vi "EXCEL 画曲线.vi"(8 "错误输入（无错误）":errorcluster, 11 "路径":path) -> (0 "error IO":errorcluster, 1 "打开时间":u32, 2 "XY图":cluster{"X":dbl, "Y":dbl}[](graph), 3 "XY图 2":cluster{"X":dbl, "Y":dbl}[](array[cluster]))   [LabVIEW 2018]
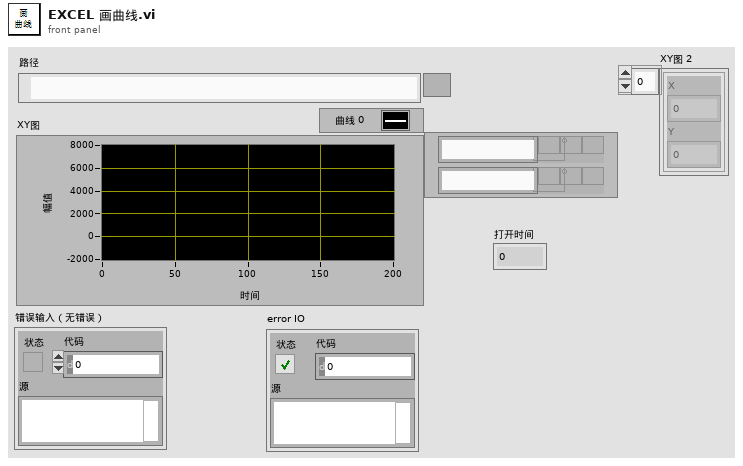
[diagram p1: front panel]
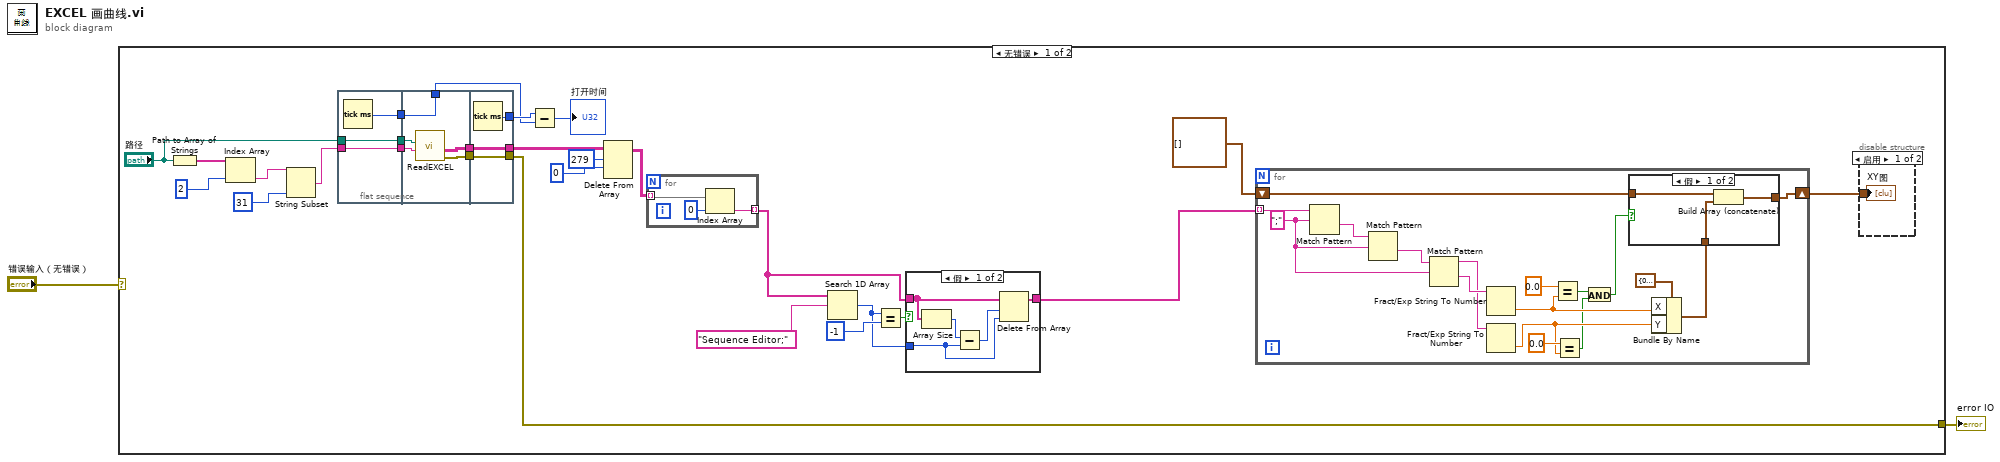
[diagram p0: block diagram]
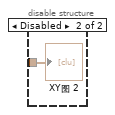
[diagram p3: hidden frame]
diagram:
  n1 = case shown="无错误" "错误输入（无错误）" {
    selector: "错误输入（无错误）" -> [_ w73]
    tunnel: [w18 w73] -> w1
    frame No Error {
      n2 = Path to Array of Strings(0:"路径") -> (2:w28:string[])  [unwired: 1 out]
      n3 = Index Array(array=w28, index=2 ("索引")) -> (element=w26:string)
      n4 = String Subset(string=w26, length (rest)=31 ("长度（剩余）")) -> (substring=w24:string)  [unwired: 1 in]
      n5 = flat-sequence {
        tunnel: w24 -> [w52]
        tunnel: "路径" -> [w53]
        tunnel: [w53] -> w9
        tunnel: [w52] -> w8
        tunnel: [w51] -> w7
        tunnel: [w56] -> w11
        tunnel: [w55] -> w10
        tunnel: w9 -> [w58]
        tunnel: w8 -> [w57]
        tunnel: w7 -> [w54]
        tunnel: [w54] -> w5
        tunnel: [w60] -> w18
        tunnel: [w61] -> w19
        tunnel: w11 -> [w61]
        tunnel: w10 -> [w60]
        tunnel: [w59] -> w6
        frame #0 {
          n6 = Tick Count (ms)() -> (millisecond timer value=w51:u32)
        }
        frame #1 {
          n7 = call "ReadEXCEL.vi"("EXCEL 标签"=w57, "路径"=w58) -> ("错误输出"=w55:errorcluster, "数据"=w56:string[][])  [unwired: 8 in]
        }
        frame #2 {
          n8 = Tick Count (ms)() -> (millisecond timer value=w59:u32)
        }
      }
      n9 = Subtract(x=w6, y=w5) -> (x-y=→"打开时间":u32)
      n10 = Delete From Array(array=w19, length=279 ("长度"), index (row)=0 ("索引 (行)")) -> (array with subset deleted=w22:string[][])  [unwired: 1 in, 1 out]
      n11 = for {
        tunnel: w22 -> [w72] mode=indexing
        tunnel: [w70] -> w15 mode=indexing
        n12 = Index Array(array=w72, index=0 ("索引")) -> (element=w70:string)
      }
      n13 = Search 1D Array(1D array=w15, element="Sequence Editor;" ("元素")) -> (index of element=w12:i32)  [unwired: 1 in]
      n14 = Equal?(x=w12, y=-1) -> (x = y?=w13:bool)
      n15 = case shown="假" w13 {
        tunnel: w15 -> [w67 w69]
        tunnel: [w68 w69] -> w14
        tunnel: w12 -> [w64 _]
        frame False {
          n16 = Array Size(array=w67) -> (size(s)=w66:i32)
          n17 = Subtract(x=w66, y=w64) -> (x-y=w65:i32)
          n18 = Delete From Array(array=w67, length=w65, index=w64) -> (array with subset deleted=w68:string[])  [unwired: 1 out]
        }
        frame True {
        }
      }
      n19 = for {
        tunnel: w14 -> [w46] mode=indexing
        shift-right: [w30] -> w23
        shift-left: cluster{"X":dbl, "Y":dbl}[] [] ("XY图") -> [w42]
        w43 = ";" ("正则表达式")
        n20 = Match Pattern(string=w46, regular expression=w43) -> (after substring=w45:string)  [unwired: 1 in, 3 out]
        n21 = Match Pattern(string=w45, regular expression=w43) -> (after substring=w44:string)  [unwired: 1 in, 3 out]
        n22 = Match Pattern(string=w44, regular expression=w43) -> (before substring=w40:string, after substring=w41:string)  [unwired: 1 in, 2 out]
        n23 = Fract/Exp String To Number(string=w41) -> (number=w38:dbl)  [unwired: 3 in, 1 out]
        n24 = Fract/Exp String To Number(string=w40) -> (number=w35:dbl)  [unwired: 3 in, 1 out]
        n25 = Equal?(x=0.0, y=w38) -> (x = y?=w33:bool)
        n26 = Equal?(x=0.0, y=w35) -> (x = y?=w34:bool)
        n27 = And(x=w33, y=w34) -> (x .and. y?=w31:bool)
        n28 = Bundle By Name(cluster=cluster{"X":dbl, "Y":dbl} {"X"=0.0, "Y"=0.0}, "X"=w38, "Y"=w35) -> (w39:cluster{"X":dbl, "Y":dbl})
        n29 = case shown="假" w31 {
          tunnel: w42 -> [w49 w50]
          tunnel: [w48 w50] -> w30
          tunnel: w39 -> [w47 _]
          frame False {
            n30 = Build Array (concatenate)(w49, w47) -> (w48:cluster{"X":dbl, "Y":dbl}[])
          }
          frame True {
          }
        }
      }
      n31 = disable-structure shown="启用" {
        disable-tunnel: w23 -> [w62 w63]
        frame Enabled {
          "XY图" <- w62
        }
        frame Disabled {
          "XY图 2" <- w63
        }
      }
    }
    frame Error {
    }
  }
  "error IO" <- w1
